vi "Generacion_contorno_3_Ejes.vi"() -> ()   [LabVIEW 2017]
uses:
  <vilib>/Motion/Express/_s/nimc.fb.straightLineMove.startStraightLineMove.axis.modeAbsolute.0.vi
  <vilib>/Motion/Express/_s/nimc.fb.contourMove.startContourMove.axis.modeFinite.vi
  <vilib>/Motion/Express/_s/nimc.fb.read.readExecutionData.axis.vi
  <vilib>/Motion/BlockNode/FB.NIMotion.xnode
  <vilib>/Motion/Express/_s/nimc.fb.contourMove.splineType.ctl
panel:
  out "Exje Z":dbl(slide)=-0.0 scale=-100.0..100.0
  in  "Stop Button":bool
  in  "Play Button":bool
  out "Eje x":dbl(slide) scale=-100.0..100.0
  out "Exje Y":dbl(slide)=-0.0 scale=-100.0..100.0
  out "XY Graph":cluster{dbl[], dbl[]}(graph)
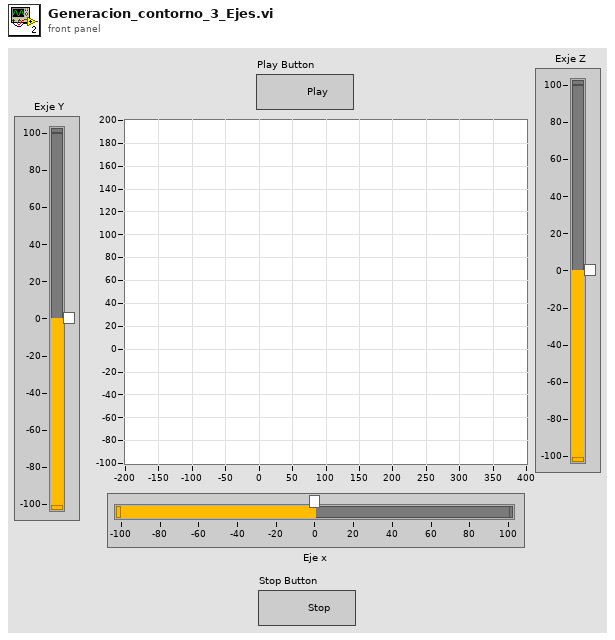
[diagram p1: front panel]
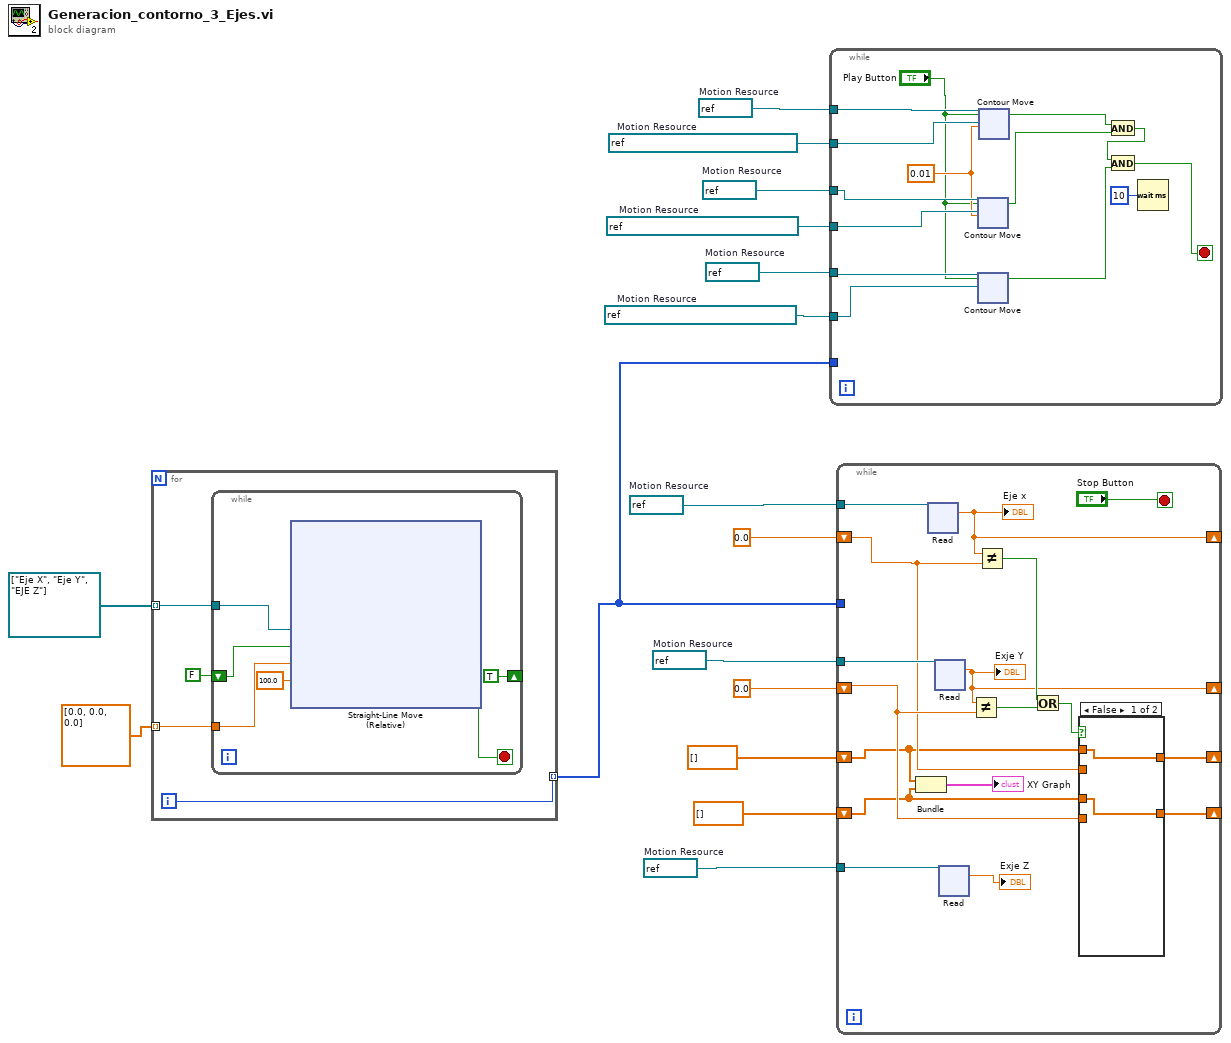
[diagram p0: block diagram]
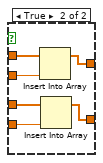
[diagram p2: hidden frame]
diagram:
  w1 = refnum<k21> "EJE Z"  # Motion Resource
  w2 = refnum<k21> "TablaZ"  # Motion Resource
  w3 = refnum<k21> "EJE Z"  # Motion Resource
  w5 = refnum<k21> "TablaX"  # Motion Resource
  w4 = refnum<k21> "TablaY"  # Motion Resource
  w6 = refnum<k21> "Eje Y"  # Motion Resource
  w8 = refnum<k21> "Eje X"  # Motion Resource
  w15 = refnum<k21> "Eje Y"  # Motion Resource
  w16 = refnum<k21> "Eje X"  # Motion Resource
  n1 = for {
    tunnel: refnum<k21>[] ["Eje X", "Eje Y", "EJE Z"] -> [w18] mode=indexing
    tunnel: dbl[] [0.0, 0.0, 0.0] -> [w19] mode=indexing
    tunnel: [w17] -> w7 mode=indexing
    i -> [w17]
    n2 = while {
      shift-right: [TRUE] -> _
      shift-left: FALSE -> [w26]
      tunnel: w19 -> [w23]
      tunnel: w18 -> [w22]
      stop <- w25 stop-if-true
      n3 = xnode "Straight-Line Move\n(Relative)"("resource"=w22, "execute"=w26, "position"=w23, "velocity"=100.0) -> ("done"=w25:bool)  [unwired: 2 in, 2 out]
    }
  }
  n4 = while {
    tunnel: w8 -> [w57]
    tunnel: w7 -> [_]
    tunnel: w6 -> [w55]
    tunnel: w5 -> [w54]
    tunnel: w4 -> [w53]
    tunnel: w3 -> [w49]
    tunnel: w2 -> [w47]
    stop <- w44 stop-if-true
    w51 = 0.01 ("interval")
    n5 = xnode "Contour Move"("resource"=w55, "execute"="Play Button", "table"=w53, "interval"=w51) -> ("done"=w52:bool)  [unwired: 2 in, 5 out]
    n6 = xnode "Contour Move"("resource"=w49, "execute"="Play Button", "table"=w47) -> ("done"=w45:bool)  [unwired: 3 in, 5 out]
    n7 = xnode "Contour Move"("resource"=w57, "execute"="Play Button", "table"=w54, "interval"=w51) -> ("done"=w56:bool)  [unwired: 2 in, 5 out]
    n8 = And(x=w56, y=w52) -> (x .and. y?=w46:bool)
    n9 = And(x=w46, y=w45) -> (x .and. y?=w44:bool)
    n10 = Wait (ms)(milliseconds to wait=u32 10) -> ()  [unwired: 1 out]
  }
  n11 = while {
    tunnel: w16 -> [w140]
    tunnel: w15 -> [w139]
    shift-right: [w128] -> _
    shift-left: 0.0 ("position") -> [w132]
    shift-right: [w127] -> _
    shift-left: 0.0 ("position") -> [w133]
    shift-right: [w135] -> _
    shift-left: dbl[] [] -> [w131]
    shift-right: [w134] -> _
    shift-left: dbl[] [] -> [w130]
    tunnel: w7 -> [_]
    tunnel: w1 -> [w124]
    stop <- "Stop Button" stop-if-true
    n12 = Bundle(w131, w130) -> (→"XY Graph":cluster{dbl[], dbl[]})  [unwired: 1 in]
    n13 = xnode "Read"("resource"=w140) -> ("position"=w128:dbl)  [unwired: 2 in, 7 out]
    "Eje x" <- w128
    n14 = xnode "Read"("resource"=w139) -> ("position"=w127:dbl)  [unwired: 2 in, 7 out]
    "Exje Y" <- w127
    n15 = xnode "Read"("resource"=w124) -> ("position"=→"Exje Z":dbl)  [unwired: 2 in, 7 out]
    n16 = Not Equal?(x=w127, y=w133) -> (x != y?=w137:bool)
    n17 = Not Equal?(x=w128, y=w132) -> (x != y?=w138:bool)
    n18 = Or(x=w138, y=w137) -> (x .or. y?=w136:bool)
    n19 = case shown="False" w136 {
      tunnel: w131 -> [w155 w161]
      tunnel: [w155 w160] -> w135
      tunnel: w130 -> [w154 w159]
      tunnel: [w154 w158] -> w134
      tunnel: w133 -> [_ w157]
      tunnel: w132 -> [_ w156]
      frame False {
      }
      frame True {
        n20 = Insert Into Array(array=w161, new element=w156) -> (w160:dbl[])  [unwired: 1 in]
        n21 = Insert Into Array(array=w159, new element=w157) -> (w158:dbl[])  [unwired: 1 in]
      }
    }
  }
